vi "AnglePIDSetup.vi"(10 "Encoder":dbl[](array[numeric]), 11 "Setpoint":dbl[](array[numeric])) -> (3 "Output":dbl[](array[numeric]))   [LabVIEW 2018]
uses:
  <vilib>/addons/control/pid/pid.llb/PID (DBL).vi
  <vilib>/addons/control/pid/NI_PID_pid.lvlib
panel:
  in  "PID gains":T1={"proportional gain (Kc)"=0.05, "integral time (Ti, min)"=0.0, "derivative time (Td, min)"=0.0} {"derivative time (Td, min)" format="%.3f"; "integral time (Ti, min)" format="%.3f"; "proportional gain (Kc)" format="%.3f"}
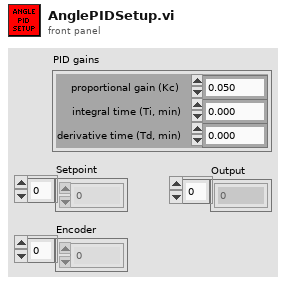
[diagram p1: front panel]
types:
  T1 = cluster{"proportional gain (Kc)":dbl, "integral time (Ti, min)":dbl, "derivative time (Td, min)":dbl}
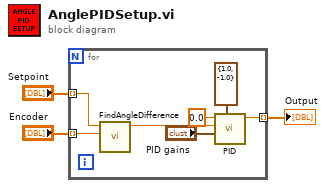
[diagram p0: block diagram]
diagram:
  n1 = for {
    tunnel: "Encoder" -> [w10] mode=indexing
    tunnel: "Setpoint" -> [w9] mode=indexing
    tunnel: [w4] -> w1 mode=indexing
    n2 = call "FindAngleDifference.vi"("AngleEncoder"=w10, "AngleSetpoint"=w9) -> ("Distance/DirectionOfTurn"=w8:dbl)  [unwired: 9 in]
    n3 = call-poly <vilib>:"PID.vi"("output range"=cluster{"output high":dbl, "output low":dbl} {"output high"=1.0, "output low"=-1.0}, "PID gains"="PID gains", "process variable"=w8, "setpoint"=0.0) -> ("output"=w4:dbl)  [unwired: 6 in, 1 out]
  }
  "Output" <- w1
